vi "Mapcluster test.vi"() -> ()   [LabVIEW 2009]
uses:
  <vilib>/Analysis/Matrix/Datatypes/RealMatrix.ctl
  <vilib>/Analysis/Matrix/NI_Matrix.lvlib
panel:
  in  "Map":T2
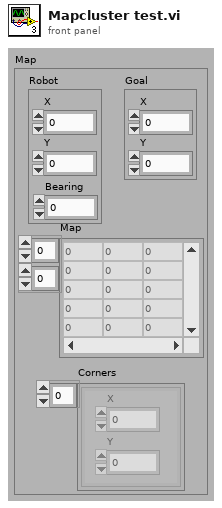
[diagram p1: front panel]
types:
  T1 = typedef "NI_Matrix.lvlib/RealMatrix.ctl" = dbl[][]
  T2 = cluster{"Robot":cluster{"X":dbl, "Y":dbl, "Bearing":dbl}, "Map":T1, "Goal":cluster{"X":dbl, "Y":dbl}, "Corners":cluster{"X":dbl, "Y":dbl}[]}
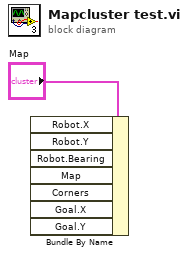
[diagram p0: block diagram]
diagram:
  n1 = Bundle By Name(cluster="Map") -> ()  [unwired: 7 in, 1 out]
